vi "CorrectInvalidProfile.vi"(0 "v0x":dbl, 1 "s3x":dbl, 2 "s0x":dbl, 3 "a1":dbl, 5 "v3x":dbl, 9 "v3y":dbl, 11 "v0y":dbl, 12 "s3y":dbl, 13 "s0y":dbl, 14 "a3":dbl) -> (6 "New v3x":dbl, 10 "New v3y":dbl)   [LabVIEW 2017]
uses:
  <vilib>/Analysis/coordinate.llb/Wrap Angle (scalar).vi
  <vilib>/Analysis/_algsub.llb/Real Vector Norm.vi
  <vilib>/Analysis/NI_AAL_Angle.lvlib
  <vilib>/Analysis/NI_AALPro.lvlib
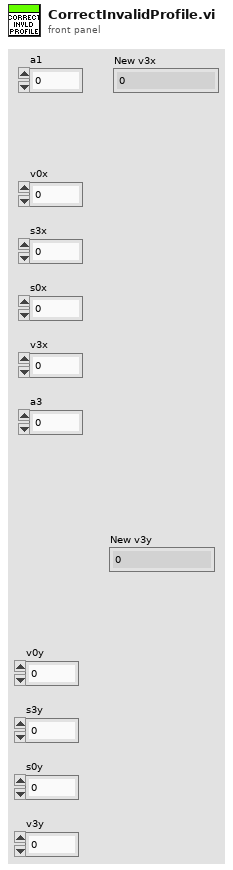
[diagram p1: front panel]
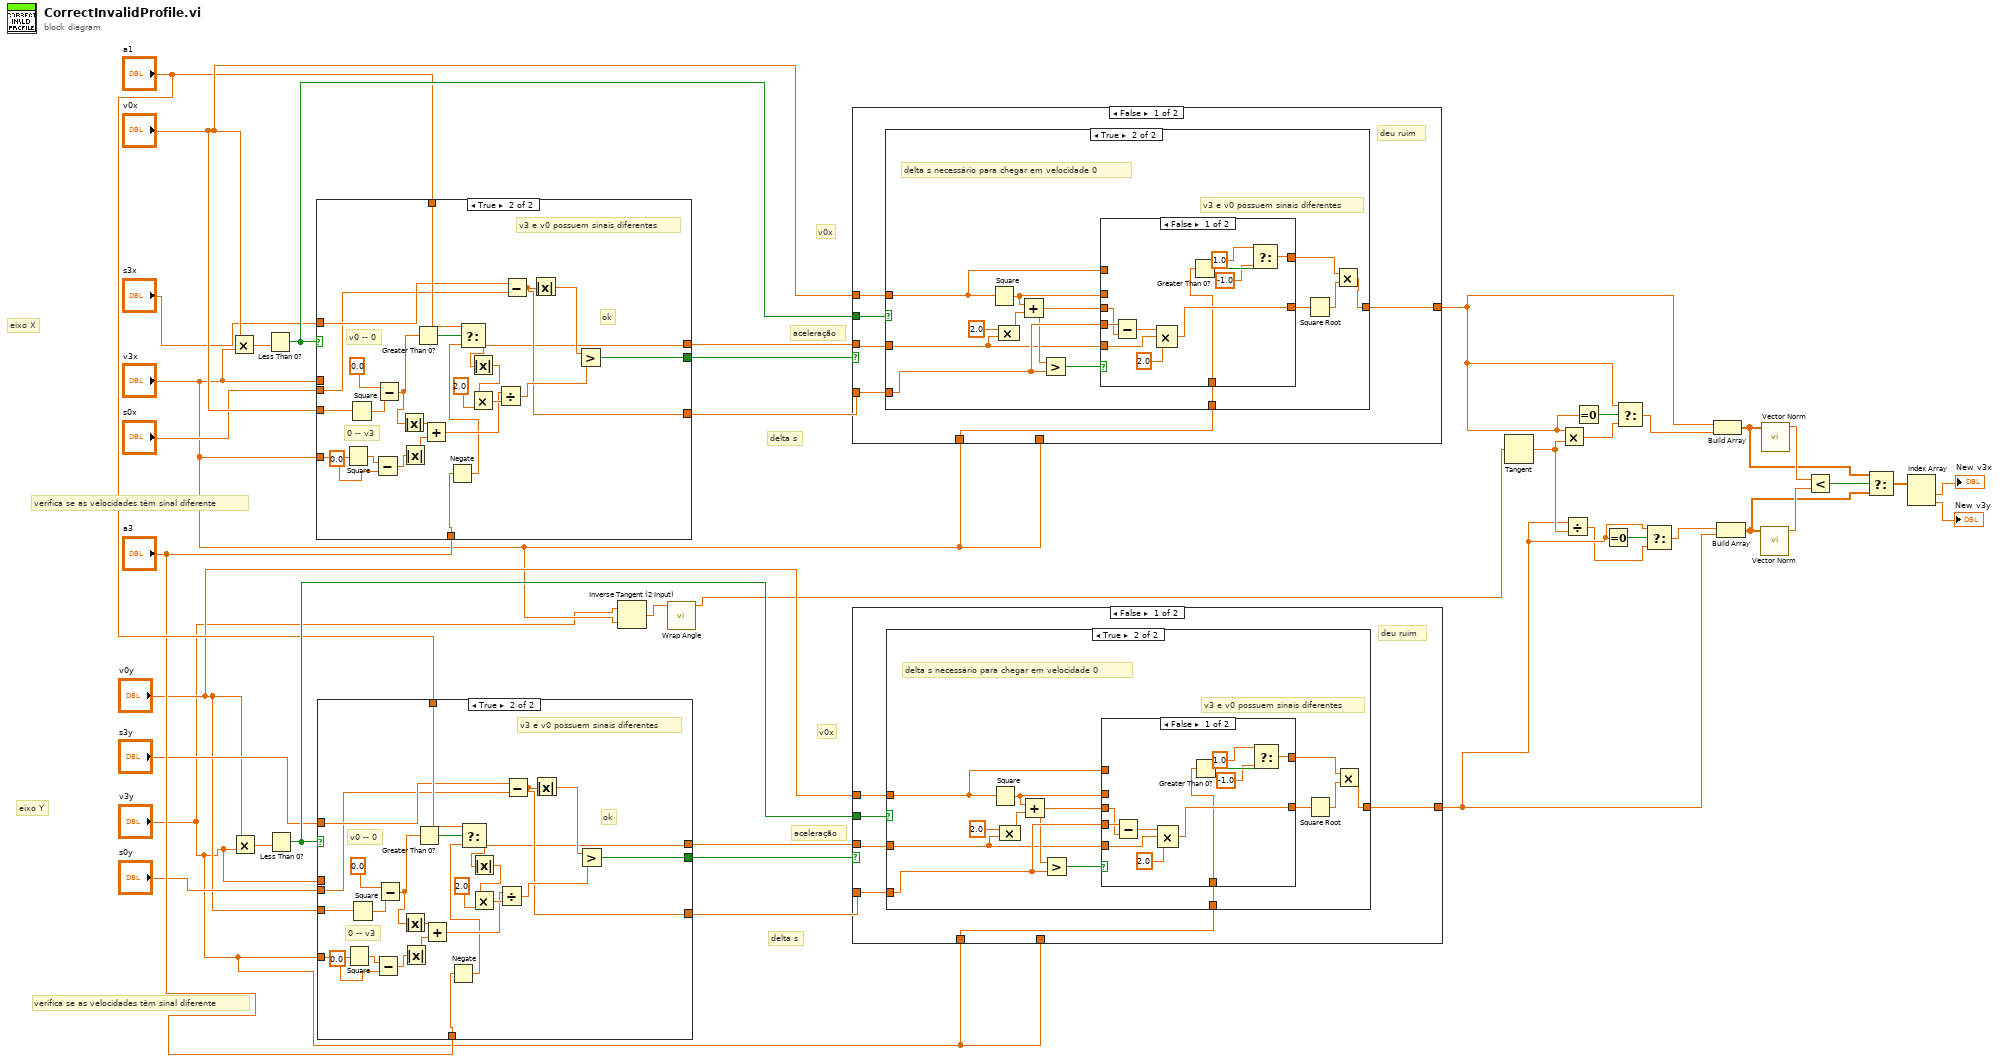
[diagram p0: block diagram]
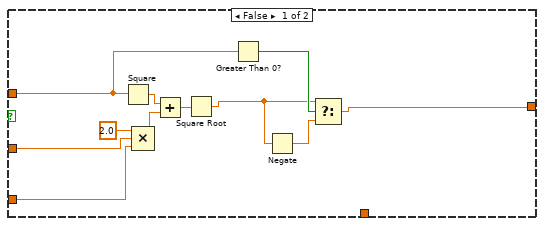
[diagram p2: hidden frame]
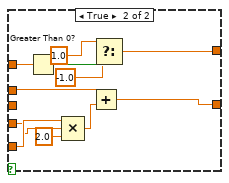
[diagram p3: hidden frame]
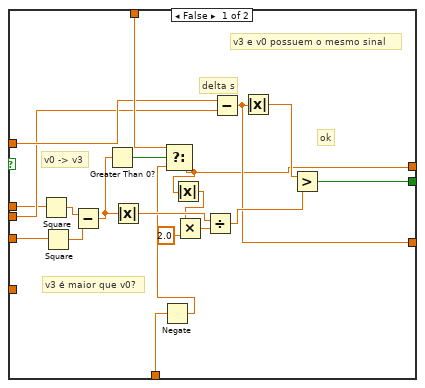
[diagram p5: hidden frame]
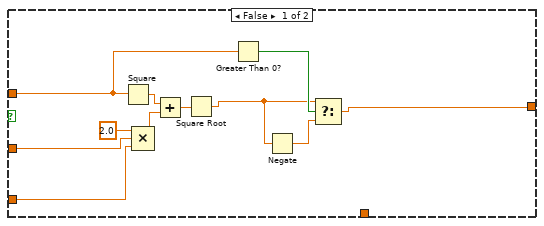
[diagram p6: hidden frame]
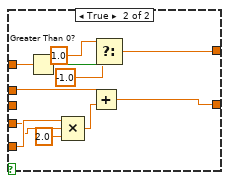
[diagram p7: hidden frame]
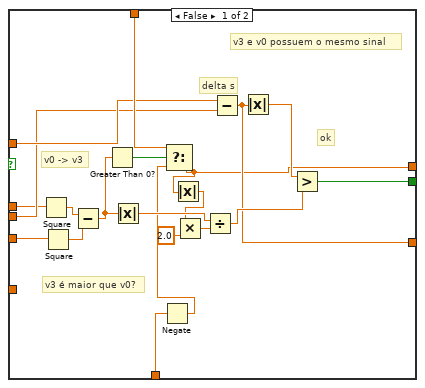
[diagram p9: hidden frame]
diagram:
  # "aceleração"
  # "v0x"
  # "verifica se as velocidades têm sinal diferente"
  # "delta s"
  # "aceleração"
  # "v0x"
  # "verifica se as velocidades têm sinal diferente"
  # "eixo Y"
  # "eixo X"
  # "delta s"
  n1 = Multiply(x="v0x", y="v3x") -> (x*y=w32:dbl)
  n2 = Multiply(x="v0y", y="v3y") -> (x*y=w27:dbl)
  n3 = Less Than 0?(x=w32) -> (x < 0?=w36:bool)
  n4 = Less Than 0?(x=w27) -> (x < 0?=w29:bool)
  n5 = case shown="True" w36 {
    tunnel: "v0x" -> [w57 w83]
    tunnel: "v3x" -> [_ w70]
    tunnel: "a3" -> [w43 w63]
    tunnel: "a1" -> [w53 w79]
    tunnel: "s3x" -> [w52 w78]
    tunnel: "s0x" -> [w51 w77]
    tunnel: [w48 w74] -> w35
    tunnel: "v3x" -> [w47 _]
    tunnel: [w41 w61] -> w38
    tunnel: [w44 w64] -> w39
    frame False {
      # "v3 é maior que v0?"
      # "v3 e v0 possuem o mesmo sinal"
      # "delta s"
      # "ok"
      # "v0 -> v3"
      n6 = Square(x=w47) -> (x^2=w59:dbl)
      n7 = Square(x=w57) -> (x^2=w58:dbl)
      n8 = Subtract(x=w59, y=w58) -> (x-y=w46:dbl)
      n9 = Greater Than 0?(x=w46) -> (x > 0?=w56:bool)
      n10 = Absolute Value(x=w46) -> (abs(x)=w45:dbl)
      n11 = Negate(x=w43) -> (-x=w42:dbl)
      n12 = Select(t=w53, s=w56, f=w42) -> (s? t:f=w41:dbl)
      n13 = Absolute Value(x=w41) -> (abs(x)=w40:dbl)
      n14 = Multiply(x=w40, y=2.0) -> (x*y=w55:dbl)
      n15 = Divide(x=w45, y=w55) -> (x/y=w49:dbl)
      n16 = Subtract(x=w52, y=w51) -> (x-y=w44:dbl)
      n17 = Absolute Value(x=w44) -> (abs(x)=w50:dbl)
      n18 = Greater?(x=w50, y=w49) -> (0:w48:bool)
    }
    frame True {
      # "v3 e v0 possuem sinais diferentes"
      # "0 -- v3"
      # "ok"
      # "v0 -- 0"
      n19 = Square(x=w70) -> (x^2=w73:dbl)
      n20 = Square(x=w83) -> (x^2=w84:dbl)
      n21 = Subtract(x=w73, y=0.0) -> (x-y=w66:dbl)
      n22 = Subtract(x=0.0, y=w84) -> (x-y=w68:dbl)
      n23 = Absolute Value(x=w68) -> (abs(x)=w67:dbl)
      n24 = Absolute Value(x=w66) -> (abs(x)=w65:dbl)
      n25 = Greater Than 0?(x=w68) -> (x > 0?=w82:bool)
      n26 = Add(x=w67, y=w65) -> (x+y=w69:dbl)
      n27 = Negate(x=w63) -> (-x=w62:dbl)
      n28 = Select(t=w79, s=w82, f=w62) -> (s? t:f=w61:dbl)
      n29 = Absolute Value(x=w61) -> (abs(x)=w60:dbl)
      n30 = Multiply(x=w60, y=2.0) -> (x*y=w81:dbl)
      n31 = Divide(x=w69, y=w81) -> (x/y=w75:dbl)
      n32 = Subtract(x=w78, y=w77) -> (x-y=w64:dbl)
      n33 = Absolute Value(x=w64) -> (abs(x)=w76:dbl)
      n34 = Greater?(x=w76, y=w75) -> (0:w74:bool)
    }
  }
  n35 = case shown="True" w29 {
    tunnel: "v0y" -> [w102 w128]
    tunnel: "v3y" -> [_ w115]
    tunnel: "a3" -> [w88 w108]
    tunnel: "a1" -> [w98 w124]
    tunnel: "s3y" -> [w97 w123]
    tunnel: "s0y" -> [w96 w122]
    tunnel: [w93 w119] -> w28
    tunnel: "v3y" -> [w92 _]
    tunnel: [w86 w106] -> w30
    tunnel: [w89 w109] -> w31
    frame False {
      # "v3 é maior que v0?"
      # "v3 e v0 possuem o mesmo sinal"
      # "delta s"
      # "ok"
      # "v0 -> v3"
      n36 = Square(x=w92) -> (x^2=w104:dbl)
      n37 = Square(x=w102) -> (x^2=w103:dbl)
      n38 = Subtract(x=w104, y=w103) -> (x-y=w91:dbl)
      n39 = Greater Than 0?(x=w91) -> (x > 0?=w101:bool)
      n40 = Absolute Value(x=w91) -> (abs(x)=w90:dbl)
      n41 = Negate(x=w88) -> (-x=w87:dbl)
      n42 = Select(t=w98, s=w101, f=w87) -> (s? t:f=w86:dbl)
      n43 = Absolute Value(x=w86) -> (abs(x)=w85:dbl)
      n44 = Multiply(x=w85, y=2.0) -> (x*y=w100:dbl)
      n45 = Divide(x=w90, y=w100) -> (x/y=w94:dbl)
      n46 = Subtract(x=w97, y=w96) -> (x-y=w89:dbl)
      n47 = Absolute Value(x=w89) -> (abs(x)=w95:dbl)
      n48 = Greater?(x=w95, y=w94) -> (0:w93:bool)
    }
    frame True {
      # "v3 e v0 possuem sinais diferentes"
      # "0 -- v3"
      # "ok"
      # "v0 -- 0"
      n49 = Square(x=w115) -> (x^2=w118:dbl)
      n50 = Square(x=w128) -> (x^2=w129:dbl)
      n51 = Subtract(x=w118, y=0.0) -> (x-y=w111:dbl)
      n52 = Subtract(x=0.0, y=w129) -> (x-y=w113:dbl)
      n53 = Absolute Value(x=w113) -> (abs(x)=w112:dbl)
      n54 = Absolute Value(x=w111) -> (abs(x)=w110:dbl)
      n55 = Greater Than 0?(x=w113) -> (x > 0?=w127:bool)
      n56 = Add(x=w112, y=w110) -> (x+y=w114:dbl)
      n57 = Negate(x=w108) -> (-x=w107:dbl)
      n58 = Select(t=w124, s=w127, f=w107) -> (s? t:f=w106:dbl)
      n59 = Absolute Value(x=w106) -> (abs(x)=w105:dbl)
      n60 = Multiply(x=w105, y=2.0) -> (x*y=w126:dbl)
      n61 = Divide(x=w114, y=w126) -> (x/y=w120:dbl)
      n62 = Subtract(x=w123, y=w122) -> (x-y=w109:dbl)
      n63 = Absolute Value(x=w109) -> (abs(x)=w121:dbl)
      n64 = Greater?(x=w121, y=w120) -> (0:w119:bool)
    }
  }
  n65 = Inverse Tangent (2 Input)(1:"v3x", 2:"v3y") -> (0:w19:dbl)
  n66 = call-poly <vilib>:"Wrap Angle.vi"("angle in"=w19) -> ("angle out"=w18:dbl)  [unwired: 9 in, 1 out]
  n67 = case shown="False" w35 {
    tunnel: w36 -> [w132 _]
    tunnel: "v0x" -> [w135 _]
    tunnel: w38 -> [w134 _]
    tunnel: w39 -> [w133 _]
    tunnel: [w131 w182] -> w7
    tunnel: "v3x" -> [_ w182]
    tunnel: "v3x" -> [w130 _]
    frame False {
      # "deu ruim"
      n68 = case shown="True" w132 {
        tunnel: w135 -> [w140 w151]
        tunnel: w134 -> [w143 w154]
        tunnel: w133 -> [w142 w156]
        tunnel: [w136 w148] -> w131
        tunnel: w130 -> [_ w147]
        frame False {
          n69 = Square(x=w140) -> (x^2=w146:dbl)
          n70 = Compound Arithmetic op=MULTIPLY(2.0 ("x"), w143, w142) -> (w145:dbl)
          n71 = Add(x=w146, y=w145) -> (x+y=w141:dbl)
          n72 = Square Root(x=w141) -> (sqrt(x)=w138:dbl)
          n73 = Greater Than 0?(x=w140) -> (x > 0?=w139:bool)
          n74 = Negate(x=w138) -> (-x=w137:dbl)
          n75 = Select(t=w138, s=w139, f=w137) -> (s? t:f=w136:dbl)
        }
        frame True {
          # "v3 e v0 possuem sinais diferentes"
          # "delta s necessário para chegar em velocidade 0"
          n76 = Square(x=w151) -> (x^2=w152:dbl)
          n77 = Compound Arithmetic op=MULTIPLY(2.0 ("x"), w154) -> (w159:dbl)
          n78 = Add(x=w152, y=w159) -> (x+y=w155:dbl)
          n79 = Greater?(x=w155, y=w156) -> (0:w157:bool)
          n80 = case shown="False" w157 {
            tunnel: w156 -> [w170 w178]
            tunnel: w155 -> [w169 _]
            tunnel: w154 -> [w167 w179]
            tunnel: [w165 w176] -> w153
            tunnel: w152 -> [_ w181]
            tunnel: w151 -> [_ w174]
            tunnel: [w161 w171] -> w150
            tunnel: w147 -> [w160 _]
            frame False {
              n81 = Subtract(x=w170, y=w169) -> (x-y=w168:dbl)
              n82 = Compound Arithmetic op=MULTIPLY(w168, w167, 2.0 ("value")) -> (w165:dbl)
              n83 = Greater Than 0?(x=w160) -> (x > 0?=w164:bool)
              n84 = Select(t=1.0, s=w164, f=-1.0) -> (s? t:f=w161:dbl)
            }
            frame True {
              n85 = Greater Than 0?(x=w174) -> (x > 0?=w175:bool)
              n86 = Compound Arithmetic op=MULTIPLY(w179, w178, 2.0 ("value")) -> (w180:dbl)
              n87 = Add(x=w181, y=w180) -> (x+y=w176:dbl)
              n88 = Select(t=1.0, s=w175, f=-1.0) -> (s? t:f=w171:dbl)
            }
          }
          n89 = Square Root(x=w153) -> (sqrt(x)=w149:dbl)
          n90 = Multiply(x=w150, y=w149) -> (x*y=w148:dbl)
        }
      }
    }
    frame True {
    }
  }
  n91 = case shown="False" w28 {
    tunnel: w29 -> [w185 _]
    tunnel: "v0y" -> [w188 _]
    tunnel: w30 -> [w187 _]
    tunnel: w31 -> [w186 _]
    tunnel: [w184 w235] -> w4
    tunnel: "v3y" -> [_ w235]
    tunnel: "v3y" -> [w183 _]
    frame False {
      # "deu ruim"
      n92 = case shown="True" w185 {
        tunnel: w188 -> [w193 w204]
        tunnel: w187 -> [w196 w207]
        tunnel: w186 -> [w195 w209]
        tunnel: [w189 w201] -> w184
        tunnel: w183 -> [_ w200]
        frame False {
          n93 = Square(x=w193) -> (x^2=w199:dbl)
          n94 = Compound Arithmetic op=MULTIPLY(2.0 ("x"), w196, w195) -> (w198:dbl)
          n95 = Add(x=w199, y=w198) -> (x+y=w194:dbl)
          n96 = Square Root(x=w194) -> (sqrt(x)=w191:dbl)
          n97 = Greater Than 0?(x=w193) -> (x > 0?=w192:bool)
          n98 = Negate(x=w191) -> (-x=w190:dbl)
          n99 = Select(t=w191, s=w192, f=w190) -> (s? t:f=w189:dbl)
        }
        frame True {
          # "v3 e v0 possuem sinais diferentes"
          # "delta s necessário para chegar em velocidade 0"
          n100 = Square(x=w204) -> (x^2=w205:dbl)
          n101 = Compound Arithmetic op=MULTIPLY(2.0 ("x"), w207) -> (w212:dbl)
          n102 = Add(x=w205, y=w212) -> (x+y=w208:dbl)
          n103 = Greater?(x=w208, y=w209) -> (0:w210:bool)
          n104 = case shown="False" w210 {
            tunnel: w209 -> [w223 w231]
            tunnel: w208 -> [w222 _]
            tunnel: w207 -> [w220 w232]
            tunnel: [w218 w229] -> w206
            tunnel: w205 -> [_ w234]
            tunnel: w204 -> [_ w227]
            tunnel: [w214 w224] -> w203
            tunnel: w200 -> [w213 _]
            frame False {
              n105 = Subtract(x=w223, y=w222) -> (x-y=w221:dbl)
              n106 = Compound Arithmetic op=MULTIPLY(w221, w220, 2.0 ("value")) -> (w218:dbl)
              n107 = Greater Than 0?(x=w213) -> (x > 0?=w217:bool)
              n108 = Select(t=1.0, s=w217, f=-1.0) -> (s? t:f=w214:dbl)
            }
            frame True {
              n109 = Greater Than 0?(x=w227) -> (x > 0?=w228:bool)
              n110 = Compound Arithmetic op=MULTIPLY(w232, w231, 2.0 ("value")) -> (w233:dbl)
              n111 = Add(x=w234, y=w233) -> (x+y=w229:dbl)
              n112 = Select(t=1.0, s=w228, f=-1.0) -> (s? t:f=w224:dbl)
            }
          }
          n113 = Square Root(x=w206) -> (sqrt(x)=w202:dbl)
          n114 = Multiply(x=w203, y=w202) -> (x*y=w201:dbl)
        }
      }
    }
    frame True {
    }
  }
  n115 = Tangent(1:w18) -> (0:w17:dbl)
  n116 = Multiply(x=w7, y=w17) -> (x*y=w6:dbl)
  n117 = Divide(x=w4, y=w17) -> (x/y=w3:dbl)
  n118 = Equal To 0?(x=w7) -> (x = 0?=w8:bool)
  n119 = Equal To 0?(x=w4) -> (x = 0?=w5:bool)
  n120 = Select(t=w7, s=w8, f=w6) -> (s? t:f=w1:dbl)
  n121 = Select(t=w4, s=w5, f=w3) -> (s? t:f=w2:dbl)
  n122 = Build Array(w7, w1) -> (w13:dbl[])
  n123 = Build Array(w2, w4) -> (w12:dbl[])
  n124 = call-poly <vilib>:"Vector Norm.vi"("Input Vector"=w12) -> ("norm"=w15:dbl)  [unwired: 9 in, 1 out]
  n125 = call-poly <vilib>:"Vector Norm.vi"("Input Vector"=w13) -> ("norm"=w16:dbl)  [unwired: 9 in, 1 out]
  n126 = Less?(x=w16, y=w15) -> (x < y?=w14:bool)
  n127 = Select(t=w13, s=w14, f=w12) -> (s? t:f=w11:dbl[])
  n128 = Index Array(array=w11) -> (element #1=→"New v3x":dbl, element #2=→"New v3y":dbl)  [unwired: 2 in]
